vi "Init.vi"(8 "error in (no error)":errorcluster, 11 "PongPanel in":refnum<class "PongPanel.lvclass">) -> (0 "error out":errorcluster, 3 "PongPanel out":refnum<class "PongPanel.lvclass">)   [LabVIEW 2019, in "RT_Game.lvlib" / "PongPanel.lvclass"]
uses:
  PongPanel.lvclass
  C:/Users/FreshBob/Dropbox/VIs/myRIO_GameConsole/RT/RT_Game/GameObject/GameObject.lvclass
  PongPanel.lvclass/PongPanel.ctl
  RT_Sprite/RT_Sprite.lvclass
  GameObject/GameObject.lvclass
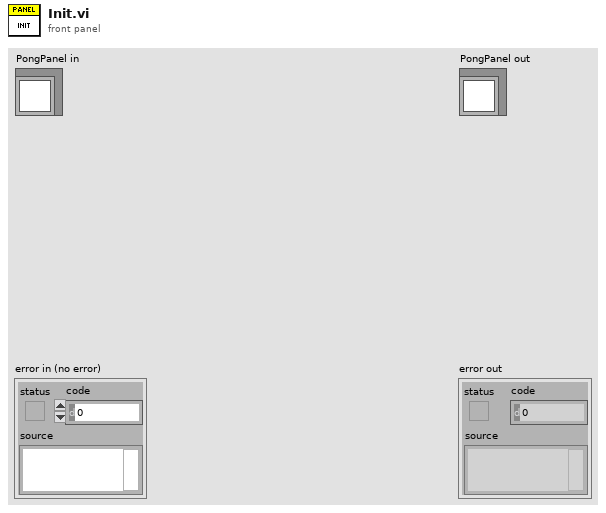
[diagram p1: front panel]
types:
  T1 = typedef "RT_Game.lvlib/Game.lvclass/Coordinate.ctl" = cluster{"x":dbl, "y":dbl}
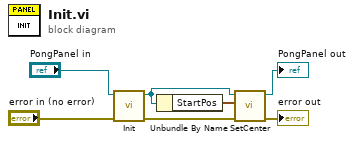
[diagram p0: block diagram]
diagram:
  n1 = call-parent "Init.vi"("error in (no error)"="error in (no error)", "RT_Sprite in"="PongPanel in") -> ("error out"=w1:errorcluster, "RT_Sprite out"=w3:refnum<class "PongPanel.lvclass">)  [unwired: 8 in]
  n2 = Unbundle By Name(w3) -> ("StartPos"=w2:T1)
  n3 = call "SetCenter.vi"("error in (no error)"=w1, "center_position"=w2, "GameObject in"=w3) -> ("error out"=→"error out":errorcluster, "GameObject out"=→"PongPanel out":refnum<class "PongPanel.lvclass">)  [unwired: 7 in]
